vi "Execute.vi"(5 "Init user event out":refnum<user-event>, 7 "user event in":refnum<user-event>, 8 "Advanced Waveform In":refnum<class "Advanced Waveform.lvclass">, 9 "Stop Message in":refnum<class "Stop Message.lvclass">, 10 "Command Queue":refnum<queue>, 11 "error in (no error)":errorcluster) -> (0 "Advanced Waveform Out":refnum<class "Advanced Waveform.lvclass">, 1 "Stop Message out":refnum<class "Stop Message.lvclass">, 2 "Stop":bool, 3 "error out":errorcluster)   [LabVIEW 2011, in "Stop Message.lvclass"]
uses:
  Stop Message.lvclass
  Advanced Waveform Class/Advanced Waveform.lvclass
  Message.lvclass
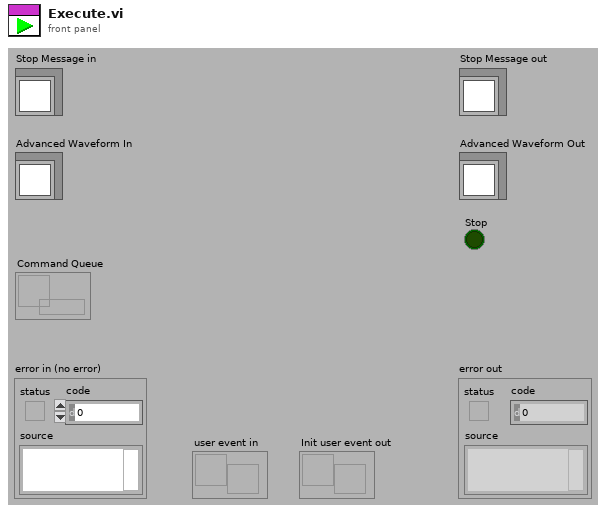
[diagram p1: front panel]
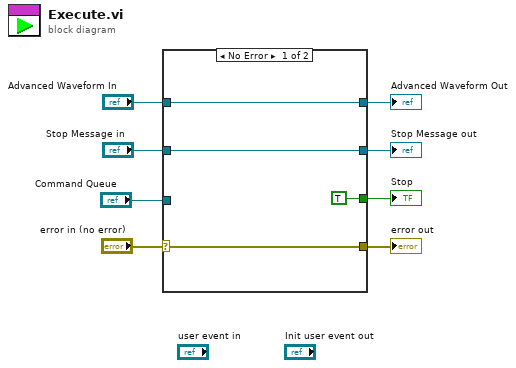
[diagram p0: block diagram]
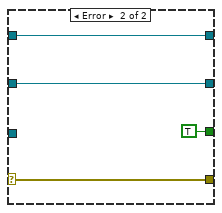
[diagram p2: hidden frame]
diagram:
  n1 = case shown="No Error" "error in (no error)" {
    selector: "error in (no error)" -> [w12 w16]
    tunnel: [w12 w16] -> w7
    tunnel: [w11 w13] -> w6
    tunnel: "Advanced Waveform In" -> [w11 w13]
    tunnel: "Stop Message in" -> [w10 w14]
    tunnel: [w10 w14] -> w3
    tunnel: "Command Queue" -> [_ _]
    tunnel: [TRUE TRUE] -> w1
    frame No Error {
    }
    frame Error {
    }
  }
  "error out" <- w7
  "Stop Message out" <- w3
  "Stop" <- w1
  "Advanced Waveform Out" <- w6
